vi "ActionVIOnCompile.vi"(8 "error in (no error)":errorcluster, 11 "Device Item Ref in":T1 format="%.0x") -> (0 "error out":errorcluster)   [LabVIEW 2017, in "Data Sharing Custom Device System Explorer.lvlib"]
uses:
  Data Sharing Custom Device System Explorer.lvlib
  <vilib>/NI Veristand/Custom Device API/Custom Device Item Ref.ctl
  Shared/Compiled.Settings.ctl
  <vilib>/NI Veristand/Custom Device API/Custom Device File Dependency.ctl
  <vilib>/NI Veristand/Custom Device API/Path Specification.ctl
  <vilib>/NI Veristand/Custom Device API/Path Type.ctl
  <vilib>/NI Veristand/Custom Device API/Custom Device Supported Target.ctl
  <vilib>/NI Veristand/Custom Device Tools/Custom Device Utility Library/NI VeriStand - Search for Item by Name.vi
  <vilib>/NI Veristand/Custom Device API/Set Item Property (Variant).vi
  <vilib>/NI VeriStand/Custom Device Tools/Custom Device Utility Library/Custom Device Utility Library.lvlib
  <vilib>/NI VeriStand/Custom Device API/Custom Device API.lvlib
  <vilib>/NI/NIVS Inline Async API/_Data Access System Explorer/Data Access System Explorer.lvlib
  Shared/Data Sharing Custom Device Shared.lvlib
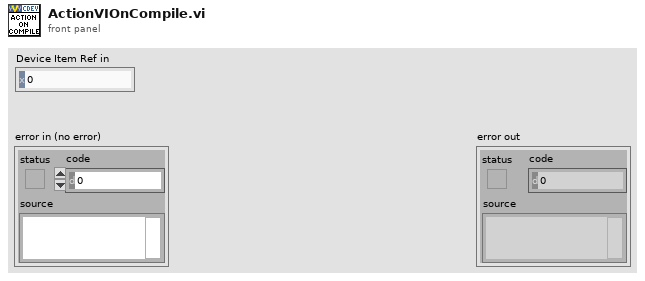
[diagram p1: front panel]
types:
  T1 = typedef "Custom Device API.lvlib/Custom Device Item Ref.ctl" = u64
  T2 = typedef "Custom Device API.lvlib/Custom Device File Dependency.ctl" = cluster{"Source":T3, "RT Destination":path, "ForceDownload?":bool, "SupportedTarget":T5, "Version":string}
  T3 = typedef "Custom Device API.lvlib/Path Specification.ctl" = cluster{"Path":path, "Type":T4}
  T4 = typedef "Custom Device API.lvlib/Path Type.ctl" = enum16{"Absolute", "To Base", "To Common Data Dir", "To Application Data Dir"}
  T5 = typedef "Custom Device API.lvlib/Custom Device Supported Target.ctl" = enum16{"All", "PharLap", "VxWorks", "Windows", "Linux_32_ARM", "Linux_x64", "PharLap & Windows", "PharLap & VxWorks", "VxWorks & Windows"}
  T6 = cluster{"Name":string, "Type":enum16{"Output/Write", "Input/Read", "Input/ReadWrite"}, "VS Refs":T1[]}
  T7 = enum16{"Output/Write", "Input/Read", "Input/ReadWrite"}
  T8 = typedef "Data Sharing Custom Device Shared.lvlib/Compiled.Settings.ctl" = cluster{"Name":string}
  T9 = typedef "Custom Device API.lvlib/Custom Device Item Info.ctl" = cluster{"Name":string, "Is Channel":bool, "GUID":string, "Is Waveform":bool}
  T10 = cluster{"Name":string, "Type":enum16{"Output/Write", "Input/Read", "Input/ReadWrite"}, "VS Refs":T1[]}[]
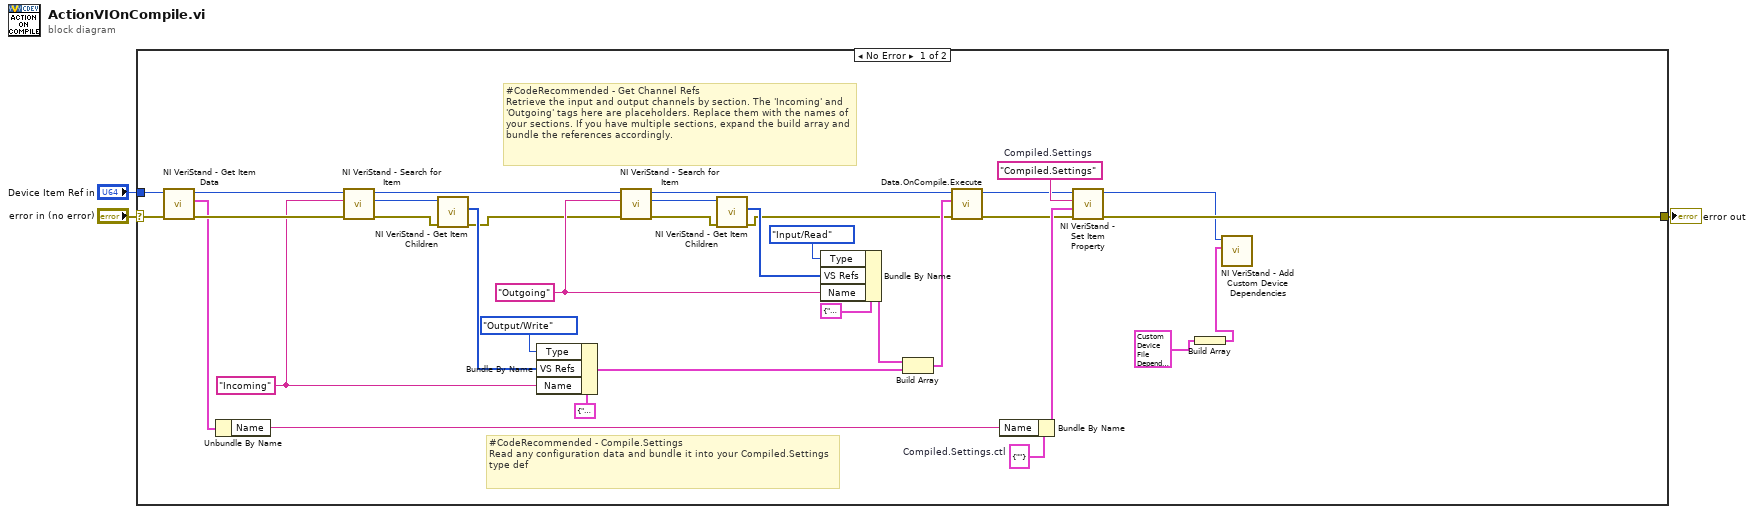
[diagram p0: block diagram]
diagram:
  n1 = case shown="No Error" "error in (no error)" {
    selector: "error in (no error)" -> [w30 w38]
    tunnel: [w31 w38] -> w2
    tunnel: "Device Item Ref in" -> [w29 _]
    frame No Error {
      w7 = T8 {"Name"=""}  # Compiled.Settings.ctl
      w22 = "Outgoing" ("Item Name")
      w24 = "Incoming" ("Item Name")
      w33 = "Compiled.Settings"  # Compiled.Settings
      # "#CodeRecommended - Get Channel Refs\nRetrieve the input and output channels by section. The 'Incoming' and 'Outgoing' tags here are placeholders. Replace them with the names of your sections. If you have multiple sections, expand the build array and bundle the references accordingly."
      # "#CodeRecommended - Compile.Settings\nRead any configuration data and bundle it into your Compiled.Settings type def"
      n2 = call <vilib>:"NI VeriStand - Get Item Data.vi"("error in (no error)"=w30, "Item Ref in"=w29) -> ("error out"=w27:errorcluster, "Item Info"=w26:T9, "Item Ref out"=w28:T1)  [unwired: 6 in, 1 out]
      n3 = Unbundle By Name(w26) -> ("Name"=w25:string)
      n4 = call-poly <vilib>:"NI VeriStand - Search for Item.vi"("error in"=w27, "Item Name"=w24, "Section Ref in"=w28) -> ("error out"=w37:errorcluster, "Item Ref"=w36:T1, "Section Ref out"=w11:T1)  [unwired: 5 in, 1 out]
      n5 = call <vilib>:"NI VeriStand - Get Item Children.vi"("error in (no error)"=w37, "Item Ref in"=w36) -> ("error out"=w10:errorcluster, "Child Refs"=w23:T1[])  [unwired: 6 in, 2 out]
      n6 = Bundle By Name(cluster=T6 {"Name"="", "Type"=enum."Output/Write", "VS Refs"=[]} ("Group"), "Type"=T7."Output/Write", "VS Refs"=w23, "Name"=w24) -> (w14:T6)
      n7 = call-poly <vilib>:"NI VeriStand - Search for Item.vi"("error in"=w10, "Item Name"=w22, "Section Ref in"=w11) -> ("error out"=w34:errorcluster, "Item Ref"=w35:T1, "Section Ref out"=w12:T1)  [unwired: 5 in, 1 out]
      n8 = call <vilib>:"NI VeriStand - Get Item Children.vi"("error in (no error)"=w34, "Item Ref in"=w35) -> ("error out"=w13:errorcluster, "Child Refs"=w18:T1[])  [unwired: 6 in, 2 out]
      n9 = Bundle By Name(cluster=T6 {"Name"="", "Type"=enum."Output/Write", "VS Refs"=[]} ("Group"), "Type"=T7."Input/Read", "VS Refs"=w18, "Name"=w22) -> (w20:T6)
      n10 = Build Array(w20, w14) -> (w17:T10)
      n11 = call <vilib>:"Data.OnCompile.Execute.vi"("error in"=w13, "VS Ref Groups"=w17, "Custom Device Ref"=w12) -> ("error out"=w9:errorcluster, "Custom Device Ref"=w8:T1)  [unwired: 7 in]
      n12 = Bundle By Name(cluster=w7, "Name"=w25) -> (w32:T8)
      n13 = call-poly <vilib>:"NI VeriStand - Set Item Property.vi"("error in (no error)"=w9, "Value"=w32, "Property Name"=w33, "Item Ref in"=w8) -> ("error out"=w31:errorcluster, "Item Ref out"=w6:T1)  [unwired: 5 in, 1 out]
      n14 = Build Array(T2 {"Source"={"Path"=path "Custom Devices/Data Sharing Custom Device/Pharlap/Data Sharing Framework Core.lvlibp", "Type"=enum."To Common Data Dir"}, "RT Destination"=path "c:/ni-rt/VeriStand/Custom Devices/Data Sharing Custom Device/Data Sharing Framework Core.lvlibp", "ForceDownload?"=TRUE, "SupportedTarget"=enum."PharLap", "Version"=""} ("Dependency")) -> (w4:T2[])
      n15 = call <vilib>:"NI VeriStand - Add Custom Device Dependencies.vi"("Dependencies"=w4, "Device Ref in"=w6) -> ()  [unwired: 8 in, 2 out]
    }
    frame Error {
    }
  }
  "error out" <- w2
